vi "Is Flat Type.vi"(8 "error in (no error)":errorcluster, 11 "LVClusterType in":refnum<class "LVClusterType.lvclass">) -> (0 "error out":errorcluster, 2 "Flat Type?":bool, 3 "LVClusterType out":refnum<class "LVClusterType.lvclass">)   [LabVIEW 2020, in "LVDataTypes.lvlib" / "LVClusterType.lvclass"]
uses:
  <vilib>/AppBuilder/Engine/WebServiceDescription/LVDataTypes/LVClusterType/LVClusterType.lvclass
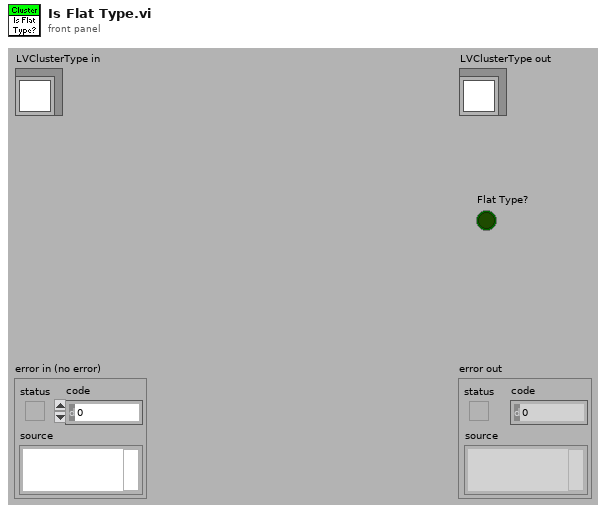
[diagram p1: front panel]
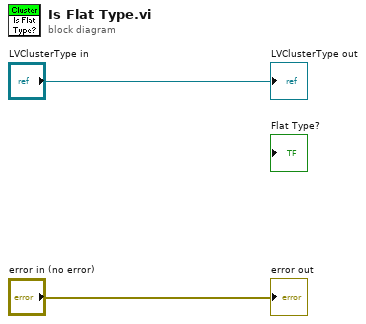
[diagram p0: block diagram]
diagram:
  "error out" <- "error in (no error)"
  "LVClusterType out" <- "LVClusterType in"
